vi "WLAN - Test - UTIL - FormatResult(vector).vi"(7 "Number":dbl[](array[numeric])) -> (8 "2nd order decimal":dbl[](array[numeric]) format="%6.1f")   [LabVIEW 2012]
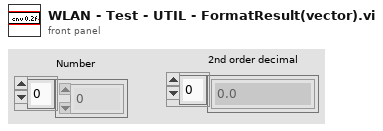
[diagram p1: front panel]
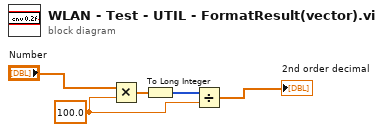
[diagram p0: block diagram]
diagram:
  w3 = 100.0 ("y")
  n1 = Multiply(x="Number", y=w3) -> (x*y=w5:dbl[])
  n2 = To Long Integer(number=w5) -> (32bit integer=w4:i32[])
  n3 = Divide(x=w4, y=w3) -> (x/y=→"2nd order decimal":dbl[])
